vi "FL_Make_Track_overlay_for_IMAQdx.vi"(5 "Full track array":T2(array[cluster]), 6 "Colors array input":u32[](array[colorbox]), 7 "Image In":T1) -> (1 "Image Out":T1)   [LabVIEW 2018]
uses:
  <vilib>/vision/Image Controls.llb/IMAQ Image.ctl
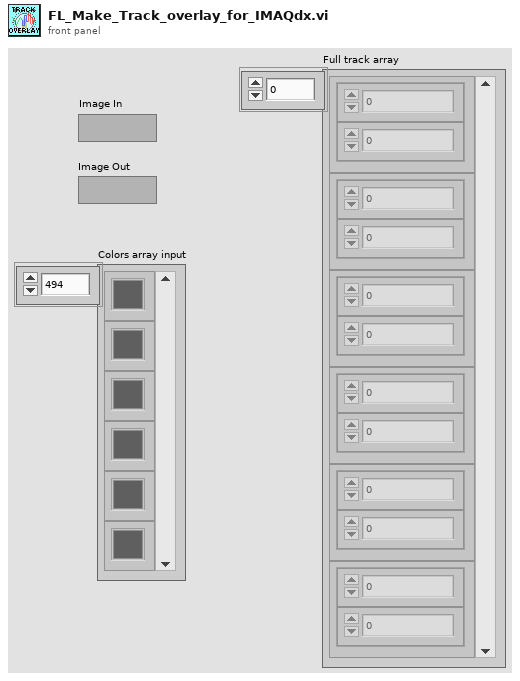
[diagram p1: front panel]
types:
  T1 = typedef "IMAQ Image.ctl" = refnum<image>
  T2 = cluster{"Numeric Control":dbl, "Numeric Control":dbl}[]
  T3 = cluster{"Numeric Control":dbl, "Numeric Control":dbl}
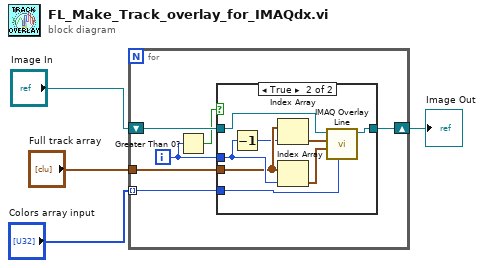
[diagram p0: block diagram]
diagram:
  n1 = for {
    tunnel: "Full track array" -> [w7]
    shift-right: [w9] -> w1
    shift-left: "Image In" -> [w10]
    tunnel: "Colors array input" -> [w8] mode=indexing
    i -> [w6]
    n2 = Greater Than 0?(x=w6) -> (x > 0?=w5:bool)
    n3 = case shown="True" w5 {
      tunnel: w10 -> [w11 w19]
      tunnel: [w11 w18] -> w9
      tunnel: w8 -> [_ w17]
      tunnel: w6 -> [_ w15]
      tunnel: w7 -> [_ w13]
      frame False {
      }
      frame True {
        n4 = Decrement(x=w15) -> (x-1=w12:i32)
        n5 = Index Array(array=w13, index=w12) -> (element=w16:T3)
        n6 = Index Array(array=w13, index=w15) -> (element=w14:T3)
        n7 = call "IMAQ Overlay Line"("Color"=w17, "End Point"=w14, "Start Point"=w16, "Image"=w19) -> ("Image Out"=w18:T1)  [unwired: 6 in, 1 out]
      }
    }
  }
  "Image Out" <- w1
